vi "GetExcelExtension.vi"(8 "error in (no error)":errorcluster, 11 "Refnum in":T1) -> (0 "error out":errorcluster, 2 "String":string, 3 "Refnum out":T1)   [LabVIEW 2013, in "main.lvlib"]
uses:
  main.lvlib
  <userlib>/Excel/excel.llb/excel Object Reference.ctl
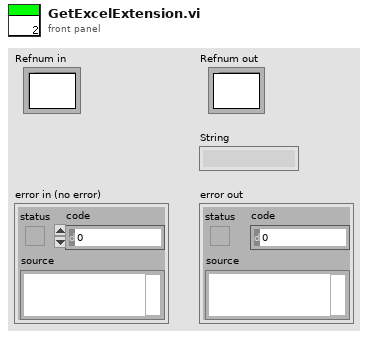
[diagram p1: front panel]
types:
  T1 = typedef "excel Object Reference.ctl" = refnum<k1>
  T2 = typedef "excel Data Members.ctl" = cluster{"Excel._Application":refnum<k7>, "Excel._Workbook":refnum<k7>, "Excel._Worksheet":refnum<k7>, "template?":bool, "location":cluster{"TopLeft":string, "RightBottom":string}, "positioning info":cluster{"direction":enum16{"right", "down"}, "gap":i32}}
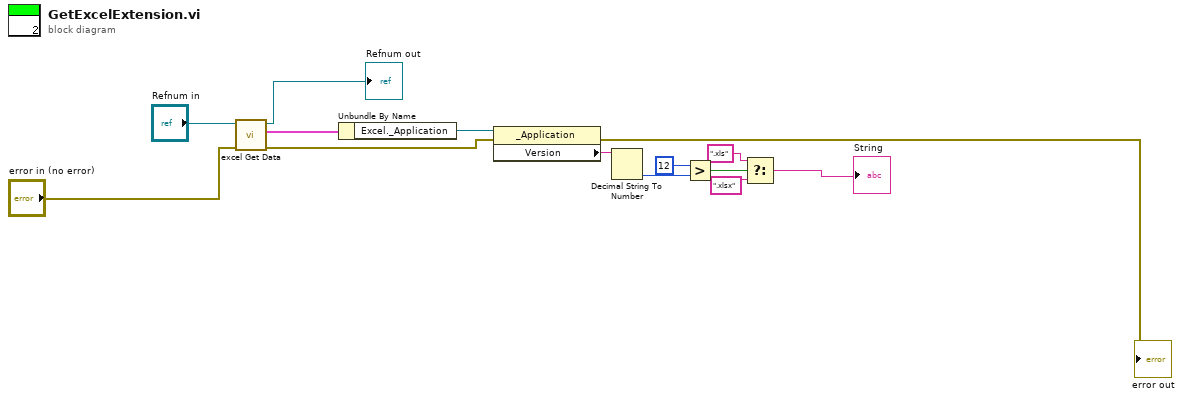
[diagram p0: block diagram]
diagram:
  n1 = call <userlib>:"excel Get Data.vi"("error in (no error)"="error in (no error)", "reference"="Refnum in") -> ("error out"=w12:errorcluster, "data"=w9:T2, "duplicate reference"=→"Refnum out":T1)  [unwired: 2 in, 1 out]
  n2 = Unbundle By Name(w9) -> ("Excel._Application"=w10:refnum<k7>)
  n3 = property class="_Application"(reference=w10, error in=w12) -> (error out=→"error out":errorcluster, "Version"=w1:string)  [unwired: 1 out]
  n4 = Decimal String To Number(string=w1) -> (number=w2:i32)  [unwired: 2 in, 1 out]
  n5 = Greater?(x=12, y=w2) -> (0:w4:bool)
  n6 = Select(t=".xls", s=w4, f=".xlsx") -> (s? t:f=→"String":string)
